vi "获取系统时间解析.vi"(11 "输入字符串":string) -> (3 "时间标识":timestamp)   [LabVIEW 2016, in "环境动力监测库.lvlib" / "空调库.lvlib"]
uses:
  <vilib>/Utility/miscctls.llb/LVDateTimeRec.ctl
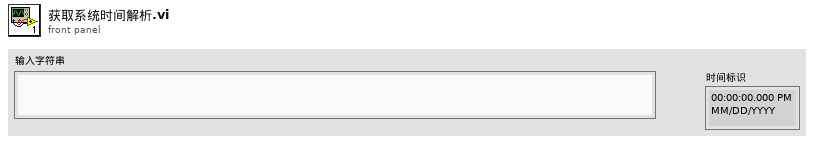
[diagram p1: front panel]
types:
  T1 = typedef "LVDateTimeRec.ctl" = cluster{"fractional second":dbl, "second":i32, "minute":i32, "hour":i32, "day of month":i32, "month":i32, "year":i32, "day of week":i32, "day of year":i32, "DST":i32}
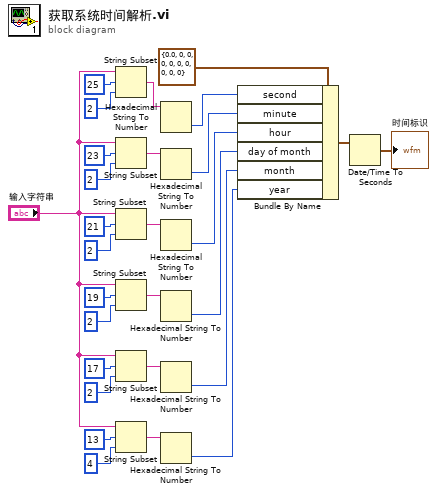
[diagram p0: block diagram]
diagram:
  n1 = String Subset(string="输入字符串", offset (0)=25 ("偏移量(0)"), length (rest)=2 ("长度（剩余）")) -> (substring=w16:string)
  n2 = String Subset(string="输入字符串", offset (0)=23 ("偏移量(0)"), length (rest)=2 ("长度（剩余）")) -> (substring=w11:string)
  n3 = String Subset(string="输入字符串", offset (0)=21 ("偏移量(0)"), length (rest)=2 ("长度（剩余）")) -> (substring=w17:string)
  n4 = String Subset(string="输入字符串", offset (0)=19 ("偏移量(0)"), length (rest)=2 ("长度（剩余）")) -> (substring=w22:string)
  n5 = String Subset(string="输入字符串", offset (0)=17 ("偏移量(0)"), length (rest)=2 ("长度（剩余）")) -> (substring=w23:string)
  n6 = String Subset(string="输入字符串", offset (0)=13 ("偏移量(0)"), length (rest)=4 ("长度（剩余）")) -> (substring=w26:string)
  n7 = Hexadecimal String To Number(string=w16) -> (number=w2:u32)  [unwired: 2 in, 1 out]
  n8 = Hexadecimal String To Number(string=w11) -> (number=w3:u32)  [unwired: 2 in, 1 out]
  n9 = Hexadecimal String To Number(string=w17) -> (number=w4:u32)  [unwired: 2 in, 1 out]
  n10 = Hexadecimal String To Number(string=w22) -> (number=w5:u32)  [unwired: 2 in, 1 out]
  n11 = Hexadecimal String To Number(string=w23) -> (number=w6:u32)  [unwired: 2 in, 1 out]
  n12 = Hexadecimal String To Number(string=w26) -> (number=w7:u32)  [unwired: 2 in, 1 out]
  n13 = Bundle By Name(cluster=T1 {"fractional second"=0.0, "second"=0, "minute"=0, "hour"=0, "day of month"=0, "month"=0, "year"=0, "day of week"=0, "day of year"=0, "DST"=0} ("日期时间记录"), "second"=w2, "minute"=w3, "hour"=w4, "day of month"=w5, "month"=w6, "year"=w7) -> (w1:T1)
  n14 = Date/Time To Seconds(2:w1) -> (0:→"时间标识":timestamp)  [unwired: 1 in]
